vi "EMI_project_v6.vi"() -> ()   [LabVIEW 2020]
uses:
  <vilib>/Instr/_visa.llb/VISA Flush IO Buffer Mask.ctl
  <vilib>/Analysis/baseanly.llb/Mean (DBL).vi
  <vilib>/Instr/_visa.llb/VISA Configure Serial Port (Instr).vi
  <vilib>/Analysis/NI_AALBase.lvlib
panel:
  out "Fader Target Level \nCH02":dbl
  out "Fader Target Level \nCH01":dbl
  out "Ref dB Level CH02":dbl
  out "Ref dB Level CH01":dbl
  out "FSR Level":dbl
  out "Voltage Average Per 5s":dbl
  out "Voltage Average Per 5s":dbl
  out "Debug":bool
  out "Auto Mix LED":bool
  in  "stop 4":bool
  in  "stop 3":bool
  out "Vol Ave Per 100 ms":dbl
  out "Vol Ave Per 100 ms":dbl
  in  "Auto Mix ON/OFF":bool
  out "Take Average CH02":bool
  out "Take Average CH01":bool
  in  "Take Average CH 01":bool
  out "Voltage Peak CH02":dynamicdata(graph)
  out "Voltage Peak CH01":dynamicdata(graph)
  in  "stop 2":bool
  out "Voltage Threshould\n CH 2":dbl
  in  "Noise Threshould \nCH02":dbl
  in  "Take Average CH 2":bool
  out "Voltage Threshould\n CH 01":dbl
  in  "Noise Threshould\n CH01":dbl
  out "Fader 02 level":dbl
  out "Fader 01 level":dbl
  out "Gain Knob 02 level":dbl
  out "Gain knob 01 level":dbl
  out "manual mode led":bool
  out "Sound Balance Mode":bool
  in  "Gain Knob 02":dbl(knob) scale=0.0..300.0
  in  "Gain Knob 01":dbl(knob) scale=0.0..300.0
  in  "Fader 02 Slider":dbl(slide) scale=0.0..10.0
  in  "Fader 01 Slider":dbl(slide) scale=0.0..10.0
  out "Fader 02 Max":dbl
  out "Fader 01 Max":dbl
  in  "Calibrate":bool
  in  "stop":bool
  in  "VISA Resource":refnum<visa-resource-name>
  in  "?":bool
  in  "Gain 02":bool
  in  "?":bool
  in  "Gain 01":bool
  in  "?":bool
  in  "Fader 02":bool
  in  "?":bool
  in  "Fader 01":bool
  # "Automation System For Analog Audio Mixers V 1.0"
  # "Calibration \nMode"
  # "Manual Mode"
  # "Sound Balance Mode"
  # "CH01"
  # "CH02"
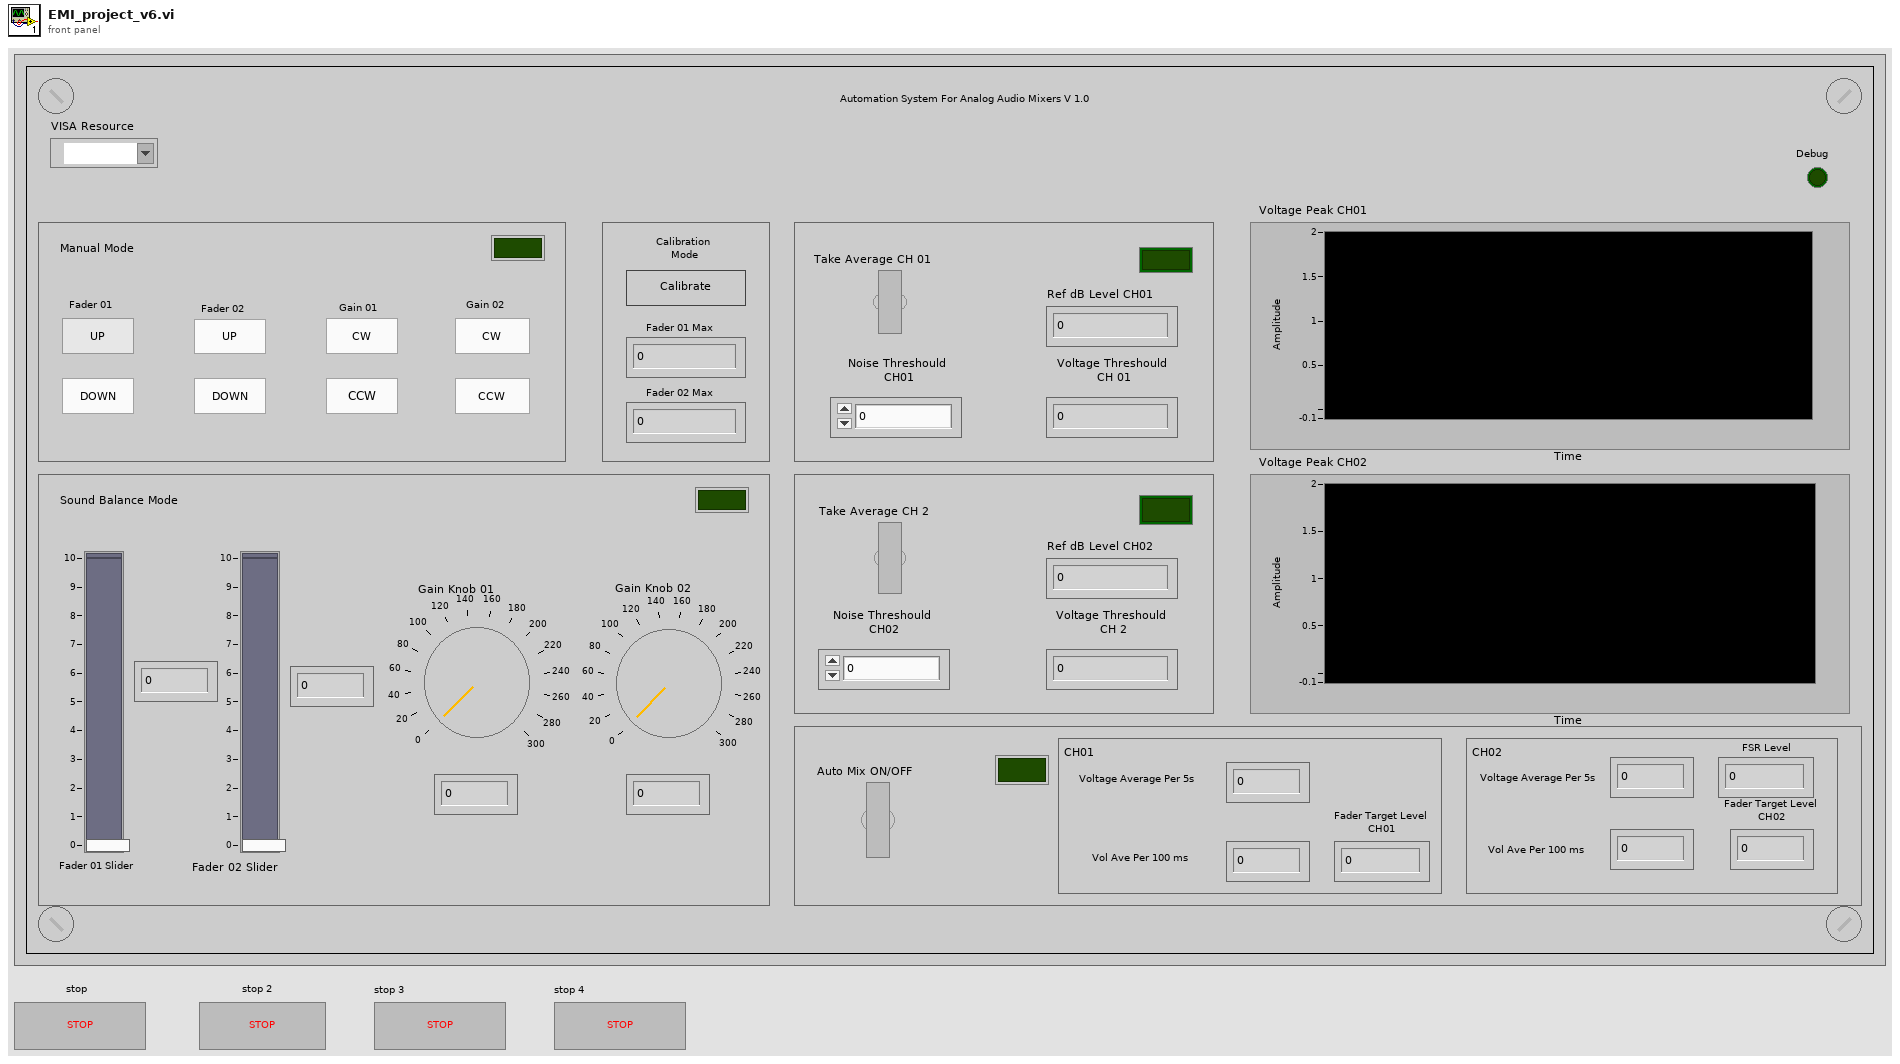
[diagram p1: front panel]
types:
  T1 = cluster{"Fader_Target_mm_1":dbl, "Fader_Target_mm_2":dbl, "Gain_Target_deg_1":dbl, "Gain_Target_deg_2":dbl}
  T2 = typedef "VISA Flush IO Buffer Mask.ctl" = u16
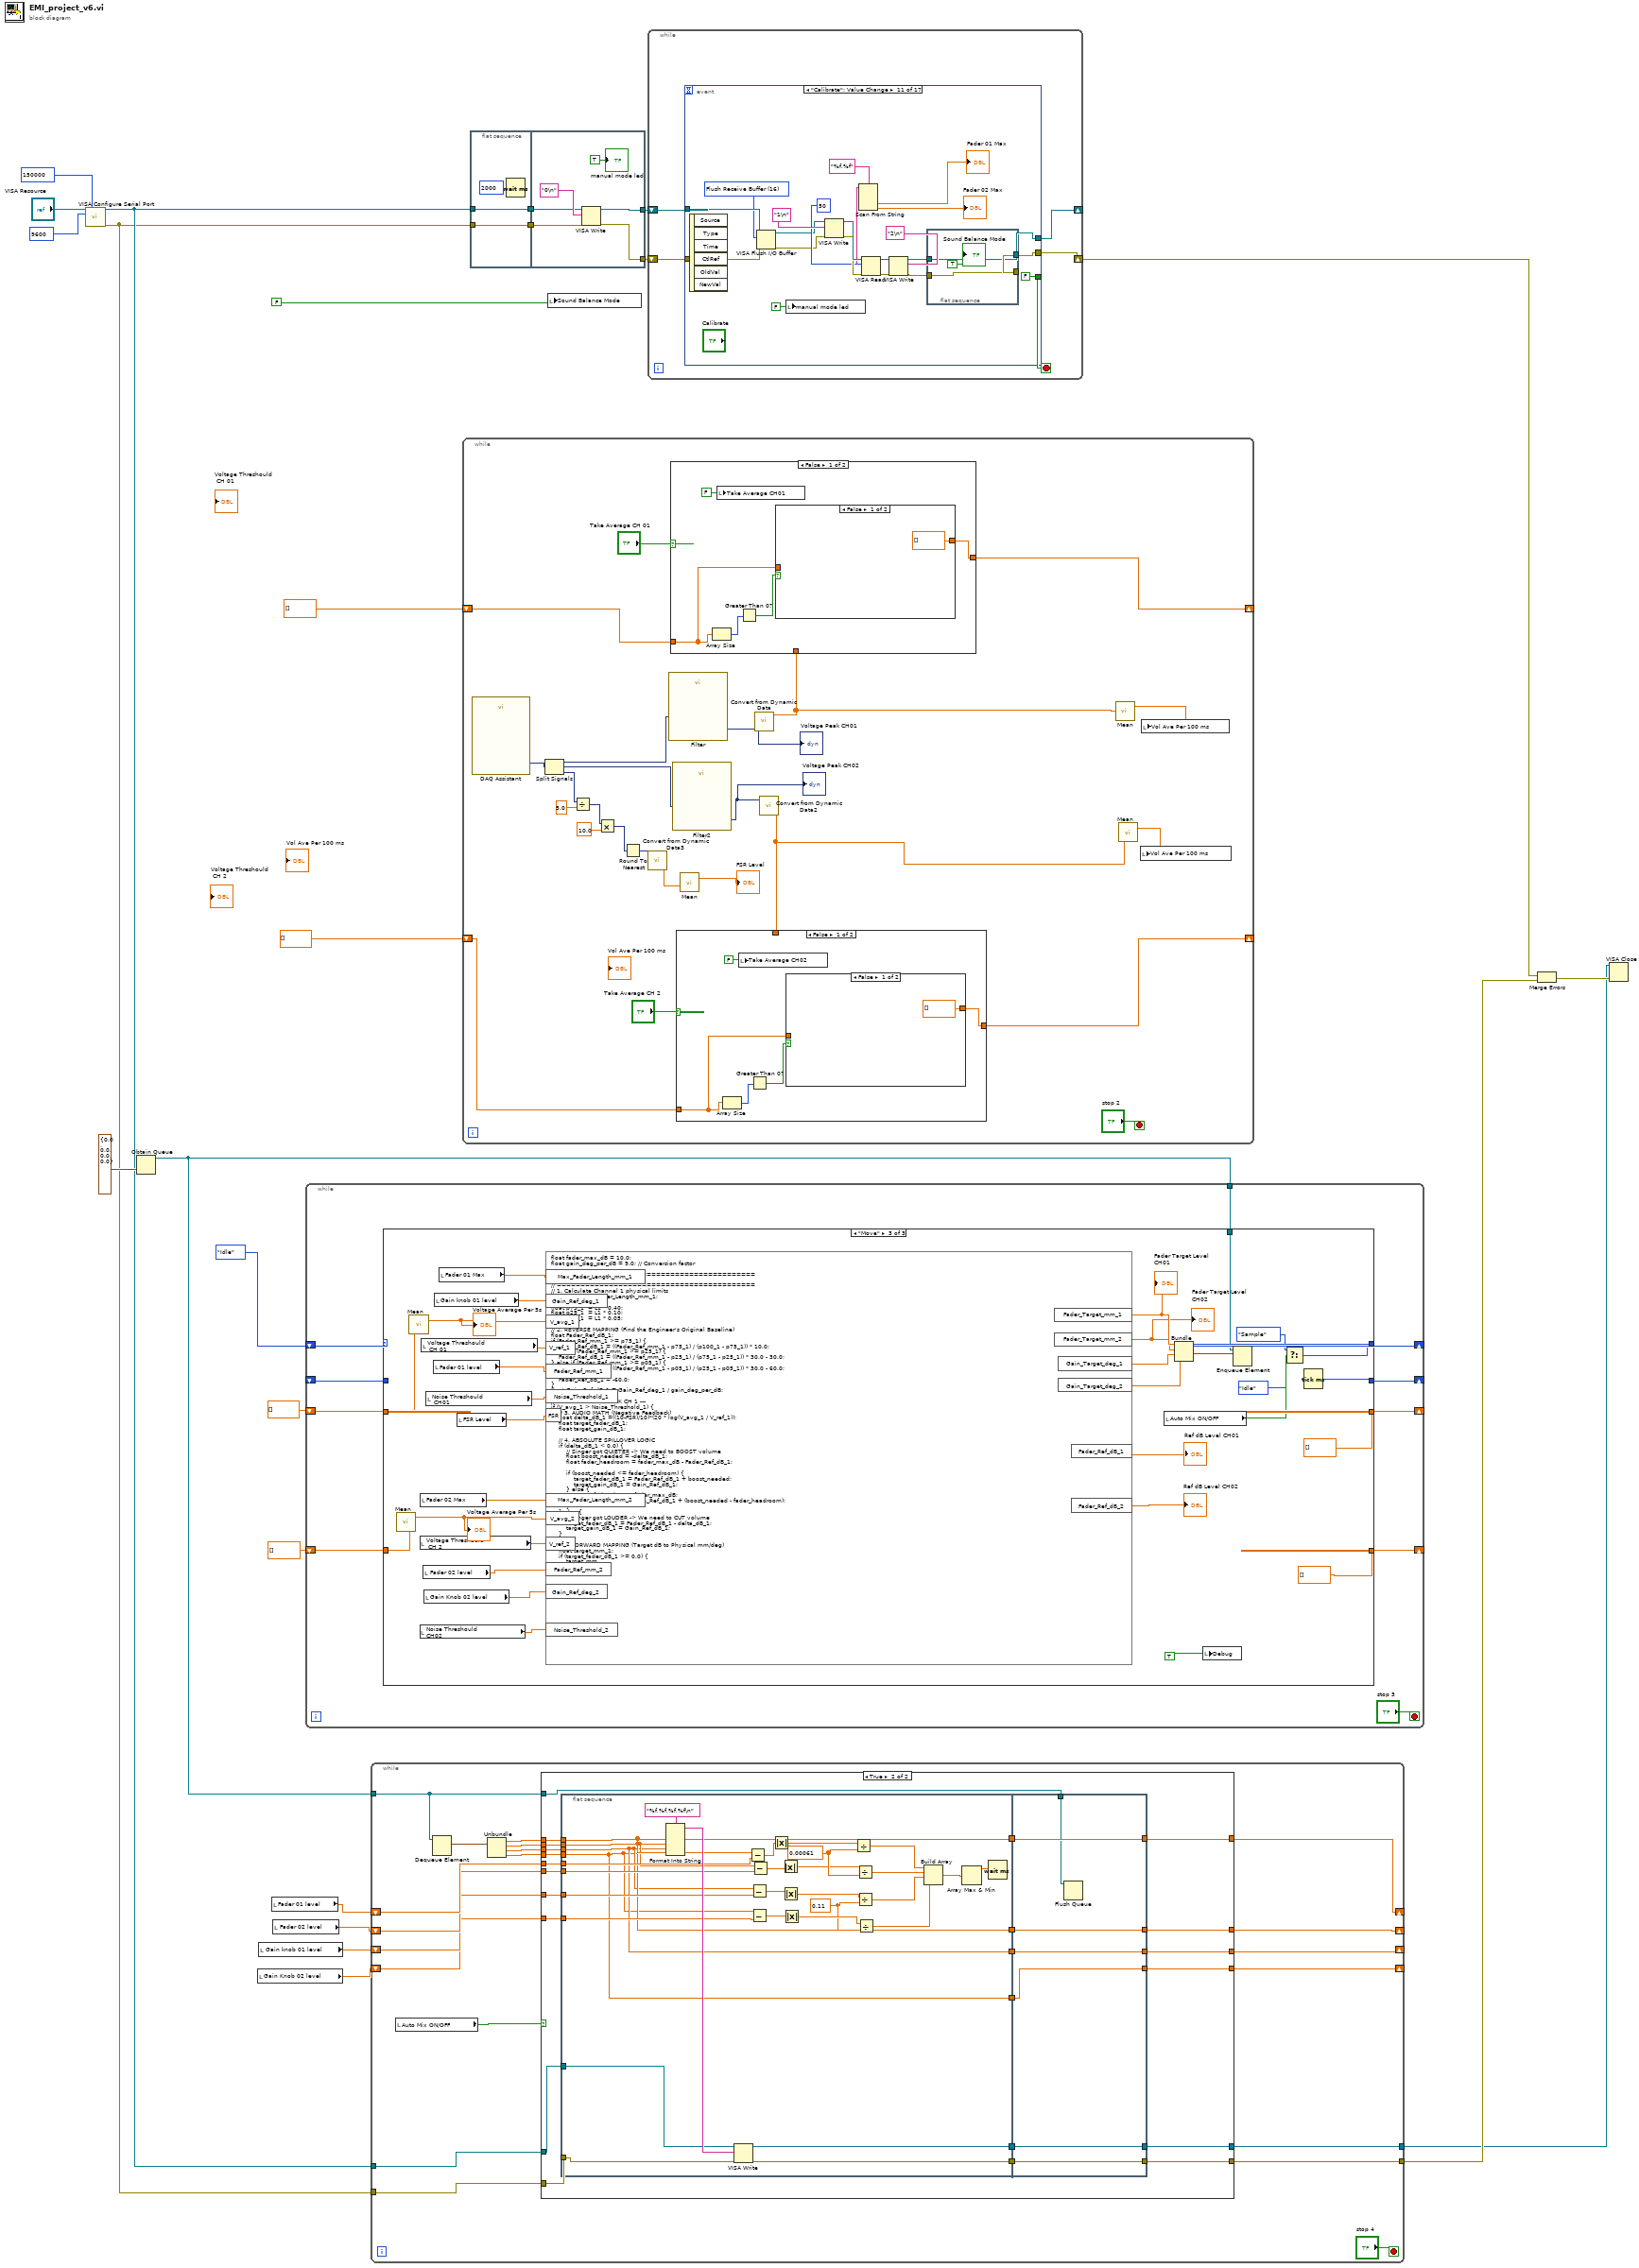
[diagram p0: block diagram]
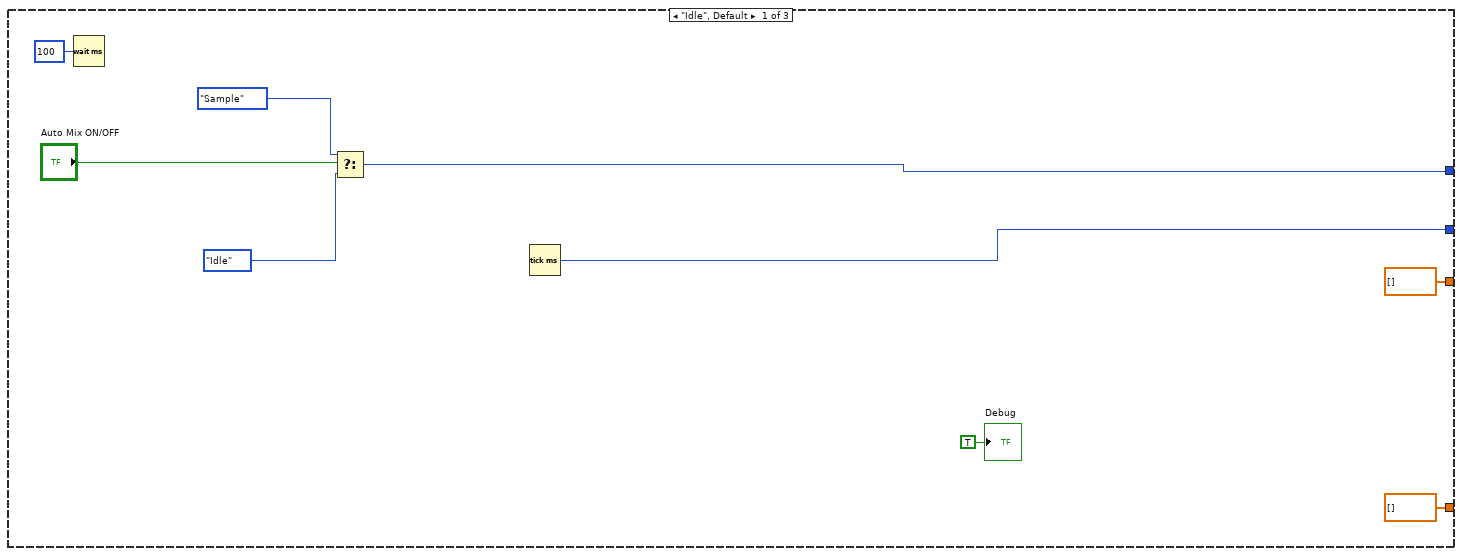
[diagram p3: hidden frame]
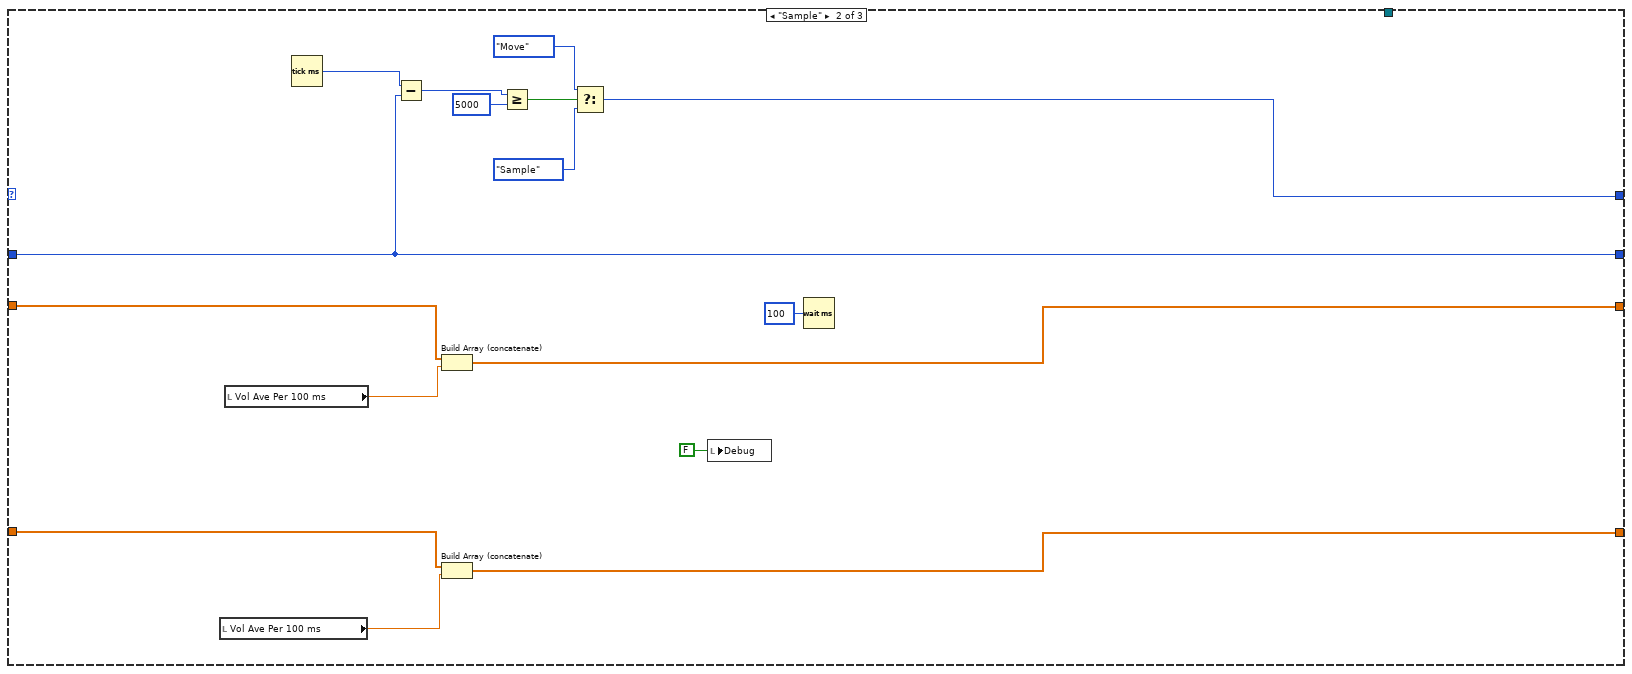
[diagram p4: hidden frame]
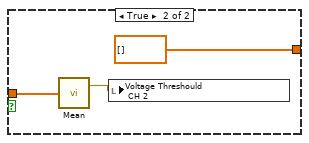
[diagram p5: hidden frame]
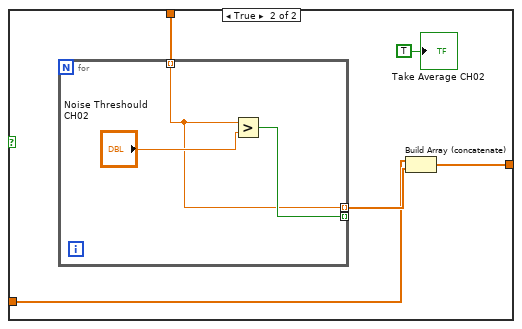
[diagram p6: hidden frame]
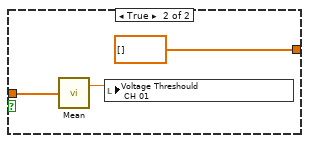
[diagram p7: hidden frame]
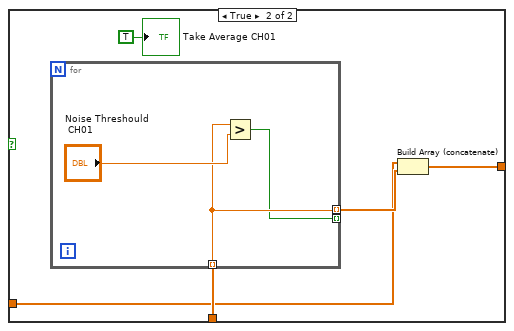
[diagram p8: hidden frame]
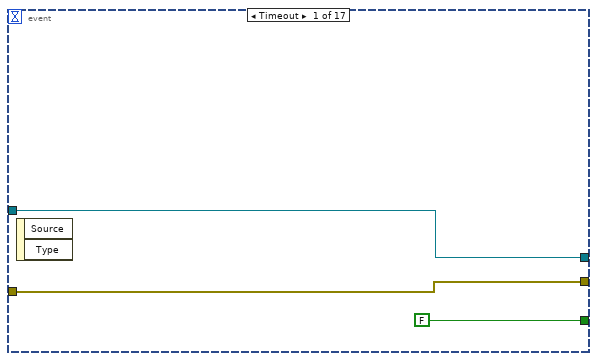
[diagram p9: hidden frame]
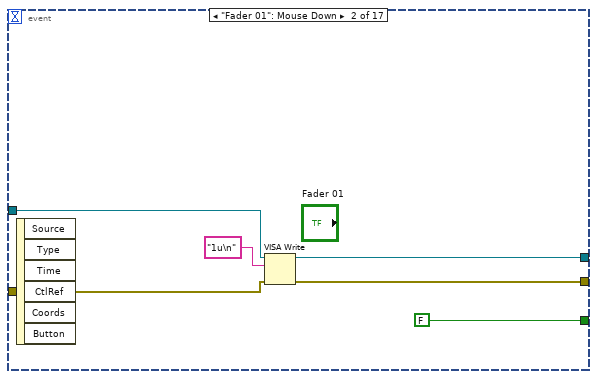
[diagram p10: hidden frame]
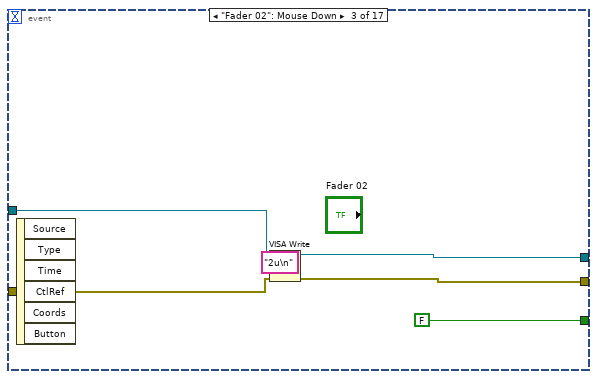
[diagram p11: hidden frame]
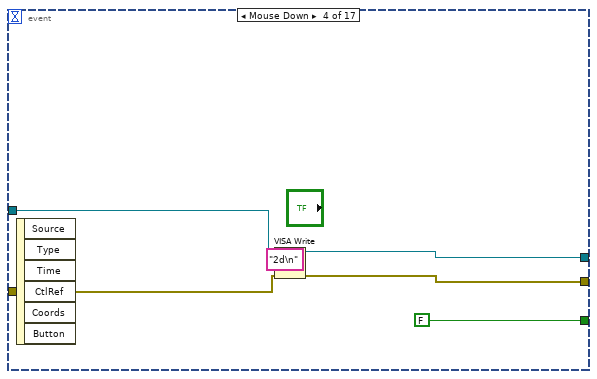
[diagram p12: hidden frame]
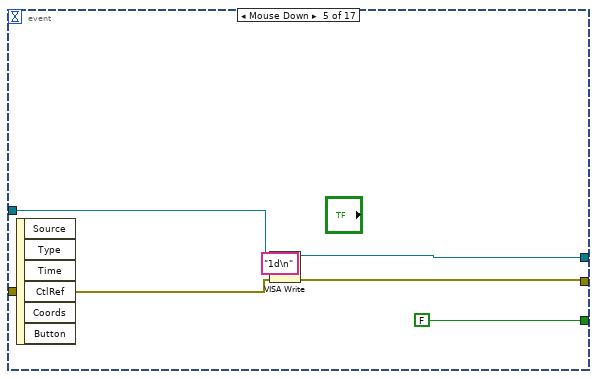
[diagram p13: hidden frame]
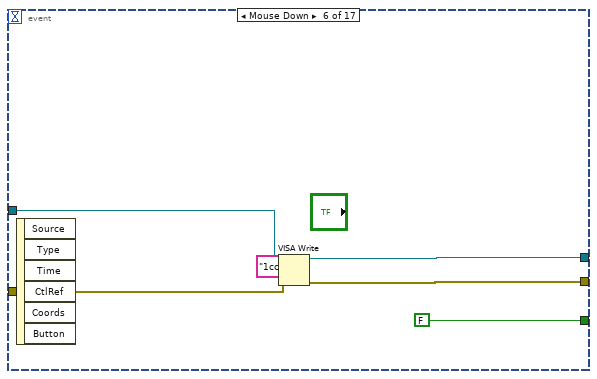
[diagram p14: hidden frame]
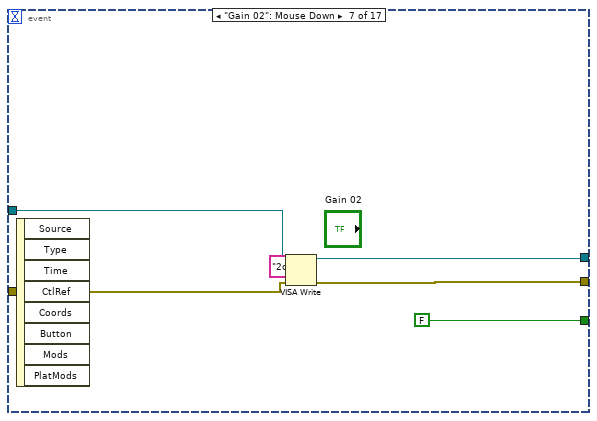
[diagram p15: hidden frame]
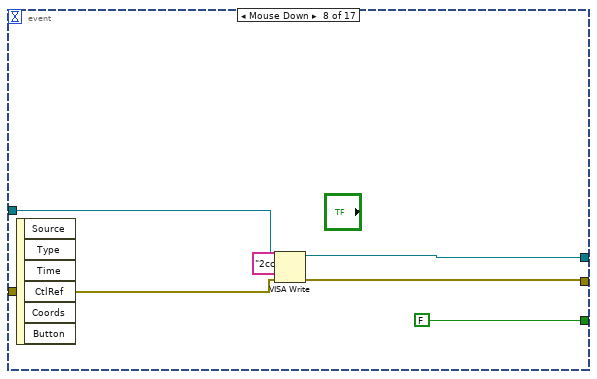
[diagram p16: hidden frame]
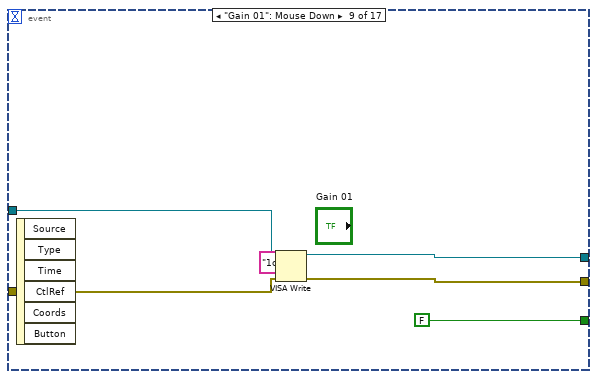
[diagram p17: hidden frame]
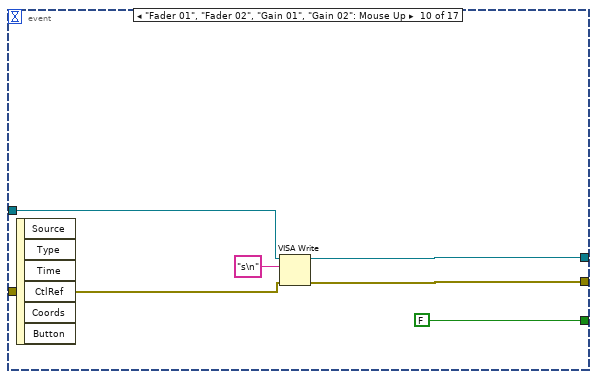
[diagram p18: hidden frame]
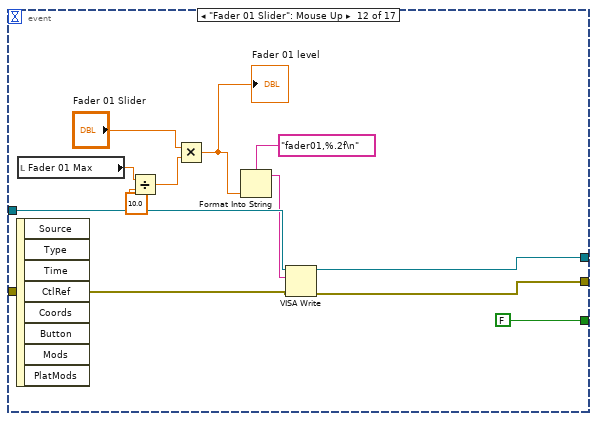
[diagram p19: hidden frame]
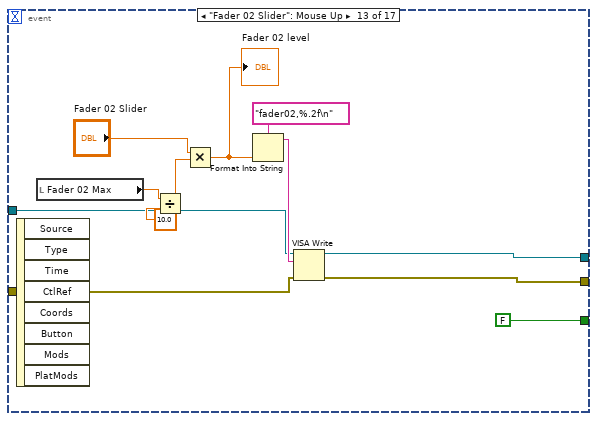
[diagram p20: hidden frame]
diagram:
  n1 = call-poly "VISA Configure Serial Port"("VISA resource name"="VISA Resource", "timeout (10sec)"=u32 150000, "baud rate (9600)"=u32 9600) -> ("VISA resource name out"=w11:refnum<visa-resource-name>, "error out"=w10:errorcluster)  [unwired: 11 in]
  n2 = Obtain Queue(element data type=T1 {"Fader_Target_mm_1"=0.0, "Fader_Target_mm_2"=0.0, "Gain_Target_deg_1"=0.0, "Gain_Target_deg_2"=0.0} ("output cluster")) -> (queue out=w12:refnum<queue>)  [unwired: 4 in, 2 out]
  n3 = local read "Gain Knob 02 level"() -> (w6:dbl)
  n4 = local read "Gain knob 01 level"() -> (w7:dbl)
  n5 = local read "Fader 01 level"() -> (w9:dbl)
  n6 = local read "Fader 02 level"() -> (w8:dbl)
  n7 = while {
    shift-right: [w34] -> _
    shift-left: enum16{"Idle", "Sample", "Move"}."Idle" -> [w35]
    shift-right: [w33] -> _
    shift-left: _ -> [w32]
    shift-right: [w30] -> _
    shift-left: dbl[] [] -> [w31]
    shift-right: [w29] -> _
    shift-left: dbl[] [] -> [w28]
    tunnel: w12 -> [w26]
    stop <- "stop 3" stop-if-true
    n8 = case shown="\"Move\"" w35 {
      tunnel: [w41 w54 w74] -> w34
      tunnel: [w36 w58 w69] -> w33
      tunnel: w32 -> [_ w58 _]
      tunnel: w31 -> [_ w53 w91]
      tunnel: [dbl[] [] w51 dbl[] []] -> w30
      tunnel: [dbl[] [] w48 dbl[] []] -> w29
      tunnel: w28 -> [_ w47 w88]
      tunnel: w26 -> [_ _ w79]
      frame "Idle", Default {
        n9 = Wait (ms)(milliseconds to wait=u32 100) -> ()  [unwired: 1 out]
        n10 = Select(t=enum16{"Idle", "Sample", "Move", "Wait"}."Sample", s="Auto Mix ON/OFF", f=enum16{"Idle", "Sample", "Move", "Wait"}."Idle") -> (s? t:f=w41:enum16{"Idle", "Sample", "Move", "Wait"})
        n11 = Tick Count (ms)() -> (millisecond timer value=w36:u32)
        "Debug" <- TRUE ("Boolean")
      }
      frame "Sample" {
        n12 = local read "Vol Ave Per 100 ms"() -> (w49:dbl)
        n13 = local read "Vol Ave Per 100 ms"() -> (w52:dbl)
        n14 = Tick Count (ms)() -> (millisecond timer value=w45:u32)
        n15 = Subtract(x=w45, y=w58) -> (x-y=w60:u32)
        n16 = Build Array (concatenate)(w53, w52) -> (w51:dbl[])
        n17 = Build Array (concatenate)(w47, w49) -> (w48:dbl[])
        n18 = Greater Or Equal?(x=w60, y=u32 5000) -> (x >= y?=w57:bool)
        n19 = Select(t=enum16{"Idle", "Sample", "Move", "Wait"}."Move", s=w57, f=enum16{"Idle", "Sample", "Move", "Wait"}."Sample") -> (s? t:f=w54:enum16{"Idle", "Sample", "Move", "Wait"})
        n20 = local write "Debug"(FALSE ("Boolean")) -> ()
        n21 = Wait (ms)(milliseconds to wait=u32 100) -> ()  [unwired: 1 out]
      }
      frame "Move" {
        n22 = call-poly <vilib>:"Mean.vi"("X"=w88) -> ("mean"=w67:dbl)  [unwired: 1 out]
        "Voltage Average Per 5s" <- w67
        n23 = call-poly <vilib>:"Mean.vi"("X"=w91) -> ("mean"=w68:dbl)  [unwired: 1 out]
        "Voltage Average Per 5s" <- w68
        n24 = local read "Voltage Threshould\n CH 2"() -> (w85:dbl)
        n25 = local read "Noise Threshould \nCH02"() -> (w71:dbl)
        n26 = local read "Fader 02 Max"() -> (w73:dbl)
        n27 = local read "Voltage Threshould\n CH 01"() -> (w86:dbl)
        n28 = local read "Fader 02 level"() -> (w82:dbl)
        n29 = local read "Gain Knob 02 level"() -> (w81:dbl)
        n30 = local read "Noise Threshould\n CH01"() -> (w72:dbl)
        n31 = local read "Fader 01 level"() -> (w84:dbl)
        n32 = local read "Gain knob 01 level"() -> (w83:dbl)
        n33 = local read "Fader 01 Max"() -> (w87:dbl)
        n34 = local read "FSR Level"() -> (w66:dbl)
        n35 = formula code="float fader_max_dB = 10.0;\nfloat gain_deg_per_dB = 9.0; // Conversion factor\n\n// ==========================================\n// CHANNEL 1 PROCESSING\n// ==========================================\n// 1. Calculate Channel 1 physical limits\nfloat L1 = Max_Fader_Length_mm_1; \nfloat p100_1 = L1;           \nfloat p75_1  = L1 * 0.40;    \nfloat p25_1  = L1 * 0.10;    \nfloat p05_1  = L1 * 0.05;    \n\n// 2. REVERSE MAPPING (Find the Engineer's Original Baseline)\nfloat Fader_Ref_dB_1;\nif (Fader_Ref_mm_1 >= p75_1) {\n    Fader_Ref_dB_1 = ((Fader_Ref_mm_1 - p75_1) / (p100_1 - p75_1)) * 10.0;\n} else if (Fader_Ref_mm_1 >= p25_1) {\n    Fader_Ref_dB_1 = ((Fader_Ref_mm_1 - p25_1) / (p75_1 - p25_1)) * 30.0 - 30.0;\n} else if (Fader_Ref_mm_1 >= p05_1) {\n    Fader_Ref_dB_1 = ((Fader_Ref_mm_1 - p05_1) / (p25_1 - p05_1)) * 30.0 - 60.0;\n} else {\n    Fader_Ref_dB_1 = -60.0; \n}\nfloat Gain_Ref_dB_1 = Gain_Ref_deg_1 / gain_deg_per_dB;\n\n// --- NOISE GATE CHECK CH 1 ---\nif (V_avg_1 > Noise_Threshold_1) {\n    // 3. AUDIO MATH (Negative Feedback)\n    float delta_dB_1 =((10-FSR)/10)*(20 * log(V_avg_1 / V_ref_1));\n    float target_fader_dB_1;\n    float target_gain_dB_1;\n\n    // 4. ABSOLUTE SPILLOVER LOGIC\n    if (delta_dB_1 < 0.0) {\n        // Singer got QUIETER -> We need to BOOST volume\n        float boost_needed = -delta_dB_1; \n        float fader_headroom = fader_max_dB - Fader_Ref_dB_1;\n        \n        if (boost_needed <= fader_headroom) {\n            target_fader_dB_1 = Fader_Ref_dB_1 + boost_needed;\n            target_gain_dB_1 = Gain_Ref_dB_1;\n        } else {\n            target_fader_dB_1 = fader_max_dB;\n            target_gain_dB_1 = Gain_Ref_dB_1 + (boost_needed - fader_headroom);\n        }\n    } else {\n        // Singer got LOUDER -> We need to CUT volume\n        target_fader_dB_1 = Fader_Ref_dB_1 - delta_dB_1;\n        target_gain_dB_1 = Gain_Ref_dB_1;\n    }\n\n    // 5. FORWARD MAPPING (Target dB to Physical mm/deg)\n    float target_mm_1;\n    if (target_fader_dB_1 >= 0.0) {\n        target_mm_1 = p75_1 + ((target_fader_dB_1 - 0.0) / 10.0) * (p100_1 - p75_1);\n    } else if (target_fader_dB_1 >= -30.0) {\n        target_mm_1 = p25_1 + ((target_fader_dB_1 - (-30.0)) / 30.0) * (p75_1 - p25_1);\n    } else if (target_fader_dB_1 >= -60.0) {\n        target_mm_1 = p05_1 + ((target_fader_dB_1 - (-60.0)) / 30.0) * (p25_1 - p05_1);\n    } else {\n        target_mm_1 = 0.0; \n    }\n\n    Fader_Target_mm_1 = target_mm_1;\n    Gain_Target_deg_1 = target_gain_dB_1 * gain_deg_per_dB; \n\n    // 6. HARDWARE SAFETY CLAMP\n    if (Gain_Target_deg_1 > 300) { Gain_Target_deg_1 = 300; }\n    if (Gain_Target_deg_1 < 0.0) { Gain_Target_deg_1 = 0.0; }\n\n} else {\n    // AUDIO IS BELOW NOISE THRESHOLD\n    // Do nothing: lock the targets to the current physical positions\n    Fader_Target_mm_1 = Fader_Ref_mm_1;\n    Gain_Target_deg_1 = Gain_Ref_deg_1;\n}\n\n\n// ==========================================\n// CHANNEL 2 PROCESSING\n// ==========================================\n// 1. Calculate Channel 2 physical limits\nfloat L2 = Max_Fader_Length_mm_2; \nfloat p100_2 = L2;           \nfloat p75_2  = L2 * 0.50;    \nfloat p25_2  = L2 * 0.10;    \nfloat p05_2  = L2 * 0.05;    \n\n// 2. REVERSE MAPPING (Find the Engineer's Original Baseline)\nfloat Fader_Ref_dB_2;\nif (Fader_Ref_mm_2 >= p75_2) {\n    Fader_Ref_dB_2 = ((Fader_Ref_mm_2 - p75_2) / (p100_2 - p75_2)) * 10.0;\n} else if (Fader_Ref_mm_2 >= p25_2) {\n    Fader_Ref_dB_2 = ((Fader_Ref_mm_2 - p25_2) / (p75_2 - p25_2)) * 30.0 - 30.0;\n} else if (Fader_Ref_mm_2 >= p05_2) {\n    Fader_Ref_dB_2 = ((Fader_Ref_mm_2 - p05_2) / (p25_2 - p05_2)) * 30.0 - 60.0;\n} else {\n    Fader_Ref_dB_2 = -60.0; \n}\nfloat Gain_Ref_dB_2 = Gain_Ref_deg_2 / gain_deg_per_dB;\n\n// --- NOISE GATE CHECK CH 2 ---\nif (V_avg_2 > Noise_Threshold_2) {\n    // 3. AUDIO MATH (Negative Feedback)\n    float delta_dB_2 = 20 * log(V_avg_1 / V_ref_1);\n    float target_fader_dB_2;\n    float target_gain_dB_2;\n\n    // 4. ABSOLUTE SPILLOVER LOGIC\n    if (delta_dB_2 < 0.0) {\n        // Singer got QUIETER -> We need to BOOST volume\n        float boost_needed = -delta_dB_2; \n        float fader_headroom = fader_max_dB - Fader_Ref_dB_2;\n        \n        if (boost_needed <= fader_headroom) {\n            target_fader_dB_2 = Fader_Ref_dB_2 + boost_needed;\n            target_gain_dB_2 = Gain_Ref_dB_2;\n        } else {\n            target_fader_dB_2 = fader_max_dB;\n            target_gain_dB_2 = Gain_Ref_dB_2 + (boost_needed - fader_headroom);\n        }\n    } else {\n        // Singer got LOUDER -> We need to CUT volume\n        target_fader_dB_2 = Fader_Ref_dB_2 - delta_dB_2;\n        target_gain_dB_2 = Gain_Ref_dB_2;\n    }\n\n    // 5. FORWARD MAPPING (Target dB to Physical mm/deg)\n    float target_mm_2;\n    if (target_fader_dB_2 >= 0.0) {\n        target_mm_2 = p75_2 + ((target_fader_dB_2 - 0.0) / 10.0) * (p100_2 - p75_2);\n    } else if (target_fader_dB_2 >= -30.0) {\n        target_mm_2 = p25_2 + ((target_fader_dB_2 - (-30.0)) / 30.0) * (p75_2 - p25_2);\n    } else if (target_fader_dB_2 >= -60.0) {\n        target_mm_2 = p05_2 + ((target_fader_dB_2 - (-60.0)) / 30.0) * (p25_2 - p05_2);\n    } else {\n        target_mm_2 = 0.0; \n    }\n\n    Fader_Target_mm_2 = target_mm_2;\n    Gain_Target_deg_2 = target_gain_dB_2 * gain_deg_per_dB; \n\n    // 6. HARDWARE SAFETY CLAMP\n    if (Gain_Target_deg_2 > 300) { Gain_Target_deg_2 = 300; }\n    if (Gain_Target_deg_2 < 0.0) { Gain_Target_deg_2 = 0.0; }\n\n} else {\n    // AUDIO IS BELOW NOISE THRESHOLD\n    // Do nothing: lock the targets to the current physical positions\n    Fader_Target_mm_2 = Fader_Ref_mm_2;\n    Gain_Target_deg_2 = Gain_Ref_deg_2;\n}"("Max_Fader_Length_mm_1"=w87, "Max_Fader_Length_mm_2"=w73, "V_avg_1"=w68, "V_ref_1"=w86, "V_avg_2"=w67, "V_ref_2"=w85, "Fader_Ref_mm_1"=w84, "Fader_Ref_mm_2"=w82, "Gain_Ref_deg_1"=w83, "Gain_Ref_deg_2"=w81, "Noise_Threshold_1"=w72, "Noise_Threshold_2"=w71, "FSR"=w66) -> ("Fader_Target_mm_1"=w63:dbl, "Fader_Target_mm_2"=w61:dbl, "Gain_Target_deg_1"=w80:dbl, "Gain_Target_deg_2"=w62:dbl, "Fader_Ref_dB_1"=→"Ref dB Level CH01":dbl, "Fader_Ref_dB_2"=→"Ref dB Level CH02":dbl)
        "Fader Target Level \nCH01" <- w63
        "Fader Target Level \nCH02" <- w61
        n36 = local read "Auto Mix ON/OFF"() -> (w77:bool)
        n37 = Bundle("Fader_Target_mm_1"=w63, "Fader_Target_mm_2"=w61, "Gain_Target_deg_1"=w80, "Gain_Target_deg_2"=w62) -> (w78:T1)  [unwired: 1 in]
        n38 = local write "Debug"(TRUE ("Boolean")) -> ()
        n39 = Enqueue Element(queue=w79, element=w78) -> ()  [unwired: 2 in, 3 out]
        n40 = Select(t=enum16{"Idle", "Sample", "Move", "Wait"}."Sample", s=w77, f=enum16{"Idle", "Sample", "Move", "Wait"}."Idle") -> (s? t:f=w74:enum16{"Idle", "Sample", "Move", "Wait"})
        n41 = Tick Count (ms)() -> (millisecond timer value=w69:u32)
      }
    }
  }
  n42 = while {
    tunnel: w12 -> [w92]
    tunnel: w11 -> [w105]
    tunnel: w10 -> [w104]
    shift-right: [w99] -> _
    shift-left: w9 -> [w103]
    shift-right: [w98] -> _
    shift-left: w8 -> [w102]
    shift-right: [w97] -> _
    shift-left: w7 -> [w101]
    shift-right: [w96] -> _
    shift-left: w6 -> [w100]
    tunnel: [w95] -> w2
    tunnel: [w94] -> w5
    stop <- "stop 4" stop-if-true
    n43 = local read "Auto Mix ON/OFF"() -> (w110:bool)
    n44 = Dequeue Element(queue=w92) -> (element=w111:T1)  [unwired: 2 in, 3 out]
    n45 = Unbundle(w111) -> ("Fader_Target_mm_1"=w109:dbl, "Fader_Target_mm_2"=w108:dbl, "Gain_Target_deg_1"=w107:dbl, "Gain_Target_deg_2"=w106:dbl)
    n46 = case shown="True" w110 {
      tunnel: w109 -> [_ w140]
      tunnel: w108 -> [_ w139]
      tunnel: w107 -> [_ w138]
      tunnel: w106 -> [_ w137]
      tunnel: w105 -> [w113 w135]
      tunnel: w104 -> [w112 w136]
      tunnel: w103 -> [w117 w134]
      tunnel: w102 -> [w116 w133]
      tunnel: w101 -> [w115 w132]
      tunnel: w100 -> [w114 w131]
      tunnel: [w117 w129] -> w99
      tunnel: [w116 w128] -> w98
      tunnel: [w115 w126] -> w97
      tunnel: [w114 w123] -> w96
      tunnel: [w113 w122] -> w95
      tunnel: [w112 w120] -> w94
      tunnel: w92 -> [_ w118]
      frame False {
      }
      frame True {
        n47 = flat-sequence {
          tunnel: w140 -> [w148]
          tunnel: w139 -> [w147]
          tunnel: w138 -> [w146]
          tunnel: w137 -> [w145]
          tunnel: w136 -> [w141]
          tunnel: w135 -> [w142]
          tunnel: w134 -> [w168]
          tunnel: w133 -> [w167]
          tunnel: w132 -> [w166]
          tunnel: w131 -> [w165]
          tunnel: [w148] -> w130
          tunnel: [w147] -> w127
          tunnel: [w146] -> w125
          tunnel: [w145] -> w124
          tunnel: [w144] -> w121
          tunnel: [w143] -> w119
          tunnel: w130 -> [w177]
          tunnel: [w177] -> w129
          tunnel: [w176] -> w128
          tunnel: w127 -> [w176]
          tunnel: [w175] -> w126
          tunnel: w125 -> [w175]
          tunnel: w124 -> [w174]
          tunnel: [w174] -> w123
          tunnel: [w173] -> w122
          tunnel: w121 -> [w173]
          tunnel: [w172] -> w120
          tunnel: w119 -> [w172]
          tunnel: w118 -> [w171]
          frame #0 {
            w151 = 0.11 ("y")
            w160 = 0.00061 ("y")
            n48 = Format Into String(format string="%f,%f,%f,%f\n", w148, w147, w146, w145) -> (resulting string=w169:string)  [unwired: 2 in, 1 out]
            n49 = VISA Write(VISA resource name=w142, write buffer=w169, error in (no error)=w141) -> (VISA resource name out=w144:refnum<visa-resource-name>, error out=w143:errorcluster)  [unwired: 1 out]
            n50 = Subtract(x=w148, y=w168) -> (x-y=w164:dbl)
            n51 = Subtract(x=w146, y=w166) -> (x-y=w162:dbl)
            n52 = Subtract(x=w145, y=w165) -> (x-y=w161:dbl)
            n53 = Subtract(x=w147, y=w167) -> (x-y=w163:dbl)
            n54 = Absolute Value(x=w164) -> (abs(x)=w159:dbl)
            n55 = Absolute Value(x=w163) -> (abs(x)=w158:dbl)
            n56 = Absolute Value(x=w162) -> (abs(x)=w157:dbl)
            n57 = Absolute Value(x=w161) -> (abs(x)=w156:dbl)
            n58 = Divide(x=w159, y=w160) -> (x/y=w155:dbl)
            n59 = Divide(x=w158, y=w160) -> (x/y=w154:dbl)
            n60 = Divide(x=w157, y=w151) -> (x/y=w153:dbl)
            n61 = Divide(x=w156, y=w151) -> (x/y=w152:dbl)
            n62 = Build Array(w155, w154, w153, w152) -> (w150:dbl[])
            n63 = Array Max & Min(array=w150) -> (max value=w149:dbl)  [unwired: 3 out]
            n64 = Wait (ms)(milliseconds to wait=w149) -> ()  [unwired: 1 out]
          }
          frame #1 {
            n65 = Flush Queue(queue=w171) -> ()  [unwired: 1 in, 3 out]
          }
        }
      }
    }
  }
  n66 = while {
    shift-right: [w197] -> _
    shift-left: dbl[] [] -> [w198]
    shift-right: [w195] -> _
    shift-left: dbl[] [] -> [w194]
    stop <- "stop 2" stop-if-true
    n67 = call "DAQ Assistant"() -> ("data"=w186:dynamicdata)  [unwired: 16 in, 3 out]
    n68 = Split Signals(w186) -> (w200:dynamicdata, w199:dynamicdata, w178:dynamicdata)  [unwired: 3 in]
    n69 = Divide(x=w178, y=5.0) -> (x/y=w183:dynamicdata)
    n70 = Multiply(x=w183, y=10.0) -> (x*y=w180:dynamicdata)
    n71 = Round To Nearest(number=w180) -> (nearest integer value=w179:dynamicdata)
    n72 = call "Convert from Dynamic Data3"("Dynamic Data Type"=w179) -> ("Array"=w184:dbl[])  [unwired: 3 in]
    n73 = call "Filter"("Signal"=w200) -> ("Filtered Signal"=w192:dynamicdata)  [unwired: 9 in, 1 out]
    "Voltage Peak CH01" <- w192
    n74 = call "Filter2"("Signal"=w199) -> ("Filtered Signal"=w191:dynamicdata)  [unwired: 9 in, 1 out]
    "Voltage Peak CH02" <- w191
    n75 = call-poly <vilib>:"Mean.vi"("X"=w184) -> ("mean"=→"FSR Level":dbl)  [unwired: 1 out]
    n76 = call "Convert from Dynamic Data"("Dynamic Data Type"=w192) -> ("Array"=w188:dbl[])  [unwired: 3 in]
    n77 = case shown="False" "Take Average CH 01" {
      tunnel: w188 -> [_ w232]
      tunnel: w198 -> [w221 w229]
      tunnel: [w220 w230] -> w197
      frame False {
        n78 = Array Size(array=w221) -> (size(s)=w223:i32)
        n79 = local write "Take Average CH01"(FALSE ("Take Average CH01")) -> ()
        n80 = Greater Than 0?(x=w223) -> (x > 0?=w222:bool)
        n81 = case shown="False" w222 {
          tunnel: w221 -> [_ w227]
          tunnel: [dbl[] [] dbl[] []] -> w220
          frame False {
          }
          frame True {
            n82 = call-poly <vilib>:"Mean.vi"("X"=w227) -> ("mean"=w226:dbl)  [unwired: 1 out]
            n83 = local write "Voltage Threshould\n CH 01"(w226) -> ()
          }
        }
      }
      frame True {
        n84 = for {
          tunnel: w232 -> [w234] mode=indexing
          tunnel: [w234] -> w231 mode=indexing if=w233
          tunnel: [w233] -> _ mode=indexing
          n85 = Greater?(x=w234, y="Noise Threshould\n CH01") -> (0:w233:bool)
        }
        n86 = Build Array (concatenate)(w229, w231) -> (w230:dbl[])
        "Take Average CH01" <- TRUE ("Take Average CH01")
      }
    }
    n87 = call "Convert from Dynamic Data2"("Dynamic Data Type"=w191) -> ("Array"=w187:dbl[])  [unwired: 3 in]
    n88 = case shown="False" "Take Average CH 2" {
      tunnel: w194 -> [w204 w214]
      tunnel: [w203 w213] -> w195
      tunnel: w187 -> [_ w212]
      frame False {
        n89 = Array Size(array=w204) -> (size(s)=w206:i32)
        n90 = local write "Take Average CH02"(FALSE ("Take Average CH02")) -> ()
        n91 = Greater Than 0?(x=w206) -> (x > 0?=w205:bool)
        n92 = case shown="False" w205 {
          tunnel: w204 -> [_ w210]
          tunnel: [dbl[] [] dbl[] []] -> w203
          frame False {
          }
          frame True {
            n93 = call-poly <vilib>:"Mean.vi"("X"=w210) -> ("mean"=w209:dbl)  [unwired: 1 out]
            n94 = local write "Voltage Threshould\n CH 2"(w209) -> ()
          }
        }
      }
      frame True {
        n95 = for {
          tunnel: [w216] -> w215 mode=indexing if=w217
          tunnel: [w217] -> _ mode=indexing
          tunnel: w212 -> [w216] mode=indexing
          n96 = Greater?(x=w216, y="Noise Threshould \nCH02") -> (0:w217:bool)
        }
        n97 = Build Array (concatenate)(w214, w215) -> (w213:dbl[])
        "Take Average CH02" <- TRUE ("Take Average CH02")
      }
    }
    n98 = call-poly <vilib>:"Mean.vi"("X"=w188) -> ("mean"=w190:dbl)  [unwired: 1 out]
    n99 = call-poly <vilib>:"Mean.vi"("X"=w187) -> ("mean"=w189:dbl)  [unwired: 1 out]
    n100 = local write "Vol Ave Per 100 ms"(w189) -> ()
    n101 = local write "Vol Ave Per 100 ms"(w190) -> ()
  }
  n102 = flat-sequence {
    tunnel: w10 -> [w237]
    tunnel: w11 -> [w238]
    tunnel: [w238] -> w21
    tunnel: [w237] -> w20
    tunnel: [w243] -> w23
    tunnel: [w242] -> w22
    tunnel: w21 -> [w241]
    tunnel: w20 -> [w240]
    frame #0 {
      n103 = Wait (ms)(milliseconds to wait=u32 2000) -> ()  [unwired: 1 out]
    }
    frame #1 {
      n104 = VISA Write(VISA resource name=w241, write buffer="0\n", error in (no error)=w240) -> (VISA resource name out=w243:refnum<visa-resource-name>, error out=w242:errorcluster)  [unwired: 1 out]
      "manual mode led" <- TRUE
    }
  }
  n105 = local write "Sound Balance Mode"(FALSE) -> ()
  n106 = while {
    shift-right: [w247] -> _
    shift-left: w23 -> [w249]
    shift-right: [w246] -> w4
    shift-left: w22 -> [w248]
    stop <- w245 stop-if-true
    n107 = event shown="[10] \"Calibrate\": Value Change" {
      selector: _ -> [_ _ _ _ _ _ _ _ _ _ _ _ _ _ _ _ _]
      dyn-events: _ -> [_ _ _ _ _ _ _ _ _ _ _ _ _ _ _ _ _]
      timeout: _ -> [_ _ _ _ _ _ _ _ _ _ _ _ _ _ _ _ _]
      tunnel: w249 -> [w252 w258 w262 w268 w276 w279 w286 w292 w298 w304 w320 w338 w349 w362 w369 w375 w393]
      tunnel: w248 -> [w251 w257 w261 w267 w275 w280 w285 w291 w297 w303 w319 w337 w348 w361 w368 w373 w392]
      tunnel: [w252 w255 w264 w270 w273 w282 w288 w294 w300 w306 w311 w334 w346 w359 w366 w374 w393] -> w247
      tunnel: [w251 w254 w263 w269 w274 w281 w287 w293 w299 w305 w308 w336 w347 w360 w367 w372 w392] -> w246
      tunnel: [FALSE FALSE FALSE FALSE FALSE FALSE FALSE FALSE FALSE FALSE FALSE FALSE FALSE FALSE FALSE FALSE TRUE] -> w245
      event Timeout {
        n108 = event-data() -> ()  [unwired: 1 in, 2 out]
      }
      event "Fader 01": Mouse Down {
        n109 = event-data() -> ()  [unwired: 1 in, 6 out]
        n110 = VISA Write(VISA resource name=w258, write buffer="1u\n", error in (no error)=w257) -> (VISA resource name out=w255:refnum<visa-resource-name>, error out=w254:errorcluster)  [unwired: 1 out]
      }
      event "Fader 02": Mouse Down {
        n111 = event-data() -> ()  [unwired: 1 in, 6 out]
        n112 = VISA Write(VISA resource name=w262, write buffer="2u\n", error in (no error)=w261) -> (VISA resource name out=w264:refnum<visa-resource-name>, error out=w263:errorcluster)  [unwired: 1 out]
      }
      event Mouse Down {
        n113 = event-data() -> ()  [unwired: 1 in, 6 out]
        n114 = VISA Write(VISA resource name=w268, write buffer="2d\n", error in (no error)=w267) -> (VISA resource name out=w270:refnum<visa-resource-name>, error out=w269:errorcluster)  [unwired: 1 out]
      }
      event Mouse Down {
        n115 = event-data() -> ()  [unwired: 1 in, 6 out]
        n116 = VISA Write(VISA resource name=w276, write buffer="1d\n", error in (no error)=w275) -> (VISA resource name out=w273:refnum<visa-resource-name>, error out=w274:errorcluster)  [unwired: 1 out]
      }
      event Mouse Down {
        n117 = event-data() -> ()  [unwired: 1 in, 6 out]
        n118 = VISA Write(VISA resource name=w279, write buffer="1ccw\n", error in (no error)=w280) -> (VISA resource name out=w282:refnum<visa-resource-name>, error out=w281:errorcluster)  [unwired: 1 out]
      }
      event "Gain 02": Mouse Down {
        n119 = event-data() -> ()  [unwired: 1 in, 8 out]
        n120 = VISA Write(VISA resource name=w286, write buffer="2cw\n", error in (no error)=w285) -> (VISA resource name out=w288:refnum<visa-resource-name>, error out=w287:errorcluster)  [unwired: 1 out]
      }
      event Mouse Down {
        n121 = event-data() -> ()  [unwired: 1 in, 6 out]
        n122 = VISA Write(VISA resource name=w292, write buffer="2ccw\n", error in (no error)=w291) -> (VISA resource name out=w294:refnum<visa-resource-name>, error out=w293:errorcluster)  [unwired: 1 out]
      }
      event "Gain 01": Mouse Down {
        n123 = event-data() -> ()  [unwired: 1 in, 6 out]
        n124 = VISA Write(VISA resource name=w298, write buffer="1cw\n", error in (no error)=w297) -> (VISA resource name out=w300:refnum<visa-resource-name>, error out=w299:errorcluster)  [unwired: 1 out]
      }
      event "Fader 01", "Fader 02", "Gain 01", "Gain 02": Mouse Up {
        n125 = event-data() -> ()  [unwired: 1 in, 6 out]
        n126 = VISA Write(VISA resource name=w304, write buffer="s\n", error in (no error)=w303) -> (VISA resource name out=w306:refnum<visa-resource-name>, error out=w305:errorcluster)  [unwired: 1 out]
      }
      event "Calibrate": Value Change {
        w316 = T2 16 items=["Flush Receive Buffer"=16, "Write Transmit Buffer to Device"=32, "Flush Receive Buffer (No I/O)"=64, "Flush Transmit Buffer"=128] ("Mask")
        n127 = event-data() -> ()  [unwired: 1 in, 6 out]
        n128 = VISA Flush I/O Buffer(VISA resource name=w320, mask (16)=w316, error in (no error)=w319) -> (VISA resource name out=w318:refnum<visa-resource-name>, error out=w317:errorcluster)
        n129 = local write "manual mode led"(FALSE ("manual mode led")) -> ()
        n130 = VISA Write(VISA resource name=w318, write buffer="1\n", error in (no error)=w317) -> (VISA resource name out=w327:refnum<visa-resource-name>, error out=w326:errorcluster)  [unwired: 1 out]
        n131 = VISA Read(VISA resource name=w327, byte count=u32 50, error in (no error)=w326) -> (VISA resource name out=w315:refnum<visa-resource-name>, read buffer=w324:string, error out=w314:errorcluster)  [unwired: 1 out]
        n132 = Scan From String(format string="%f,%f", input string=w324) -> (output 1=→"Fader 01 Max":dbl, output 2=→"Fader 02 Max":dbl)  [unwired: 4 in, 3 out]
        n133 = VISA Write(VISA resource name=w315, write buffer="2\n", error in (no error)=w314) -> (VISA resource name out=w310:refnum<visa-resource-name>, error out=w309:errorcluster)  [unwired: 1 out]
        n134 = flat-sequence {
          tunnel: [w330] -> w311
          tunnel: w310 -> [w330]
          tunnel: w309 -> [w329]
          tunnel: [w329] -> w308
          frame #0 {
            "Sound Balance Mode" <- TRUE
          }
        }
      }
      event "Fader 01 Slider": Mouse Up {
        n135 = event-data() -> ()  [unwired: 1 in, 8 out]
        n136 = local read "Fader 01 Max"() -> (w342:dbl)
        n137 = Divide(x=w342, y=10.0) -> (x/y=w339:dbl)
        n138 = Multiply(x="Fader 01 Slider", y=w339) -> (x*y=w332:dbl)
        "Fader 01 level" <- w332
        n139 = Format Into String(format string="fader01,%.2f\n", w332) -> (resulting string=w333:string)  [unwired: 2 in, 1 out]
        n140 = VISA Write(VISA resource name=w338, write buffer=w333, error in (no error)=w337) -> (VISA resource name out=w334:refnum<visa-resource-name>, error out=w336:errorcluster)  [unwired: 1 out]
      }
      event "Fader 02 Slider": Mouse Up {
        n141 = event-data() -> ()  [unwired: 1 in, 8 out]
        n142 = local read "Fader 02 Max"() -> (w355:dbl)
        n143 = Divide(x=w355, y=10.0) -> (x/y=w352:dbl)
        n144 = Multiply(x="Fader 02 Slider", y=w352) -> (x*y=w344:dbl)
        "Fader 02 level" <- w344
        n145 = Format Into String(format string="fader02,%.2f\n", w344) -> (resulting string=w350:string)  [unwired: 2 in, 1 out]
        n146 = VISA Write(VISA resource name=w349, write buffer=w350, error in (no error)=w348) -> (VISA resource name out=w346:refnum<visa-resource-name>, error out=w347:errorcluster)  [unwired: 1 out]
      }
      event "Gain Knob 01": Mouse Up {
        n147 = event-data() -> ()  [unwired: 1 in, 8 out]
        n148 = Format Into String(format string="gain01,%.2f\n", "Gain Knob 01") -> (resulting string=w358:string)  [unwired: 2 in, 1 out]
        n149 = VISA Write(VISA resource name=w362, write buffer=w358, error in (no error)=w361) -> (VISA resource name out=w359:refnum<visa-resource-name>, error out=w360:errorcluster)  [unwired: 1 out]
        "Gain knob 01 level" <- "Gain Knob 01"
      }
      event "Gain Knob 02": Mouse Up {
        n150 = event-data() -> ()  [unwired: 1 in, 8 out]
        n151 = Format Into String(format string="gain02,%.2f\n", "Gain Knob 02") -> (resulting string=w370:string)  [unwired: 2 in, 1 out]
        n152 = VISA Write(VISA resource name=w369, write buffer=w370, error in (no error)=w368) -> (VISA resource name out=w366:refnum<visa-resource-name>, error out=w367:errorcluster)  [unwired: 1 out]
        "Gain Knob 02 level" <- "Gain Knob 02"
      }
      event "Auto Mix ON/OFF": Value Change {
        n153 = event-data() -> ()  [unwired: 1 in, 6 out]
        n154 = local read "Auto Mix ON/OFF"() -> (w377:bool)
        n155 = case shown="False" w377 {
          tunnel: w375 -> [w381 w391]
          tunnel: [w383 w390] -> w374
          tunnel: w373 -> [w384 w389]
          tunnel: [w382 w388] -> w372
          frame False {
            n156 = local write "Sound Balance Mode"(TRUE ("Sound Balance Mode")) -> ()
            n157 = VISA Write(VISA resource name=w381, write buffer="2\n", error in (no error)=w384) -> (VISA resource name out=w383:refnum<visa-resource-name>, error out=w382:errorcluster)  [unwired: 1 out]
            n158 = local write "Auto Mix LED"(FALSE ("Auto Mix LED")) -> ()
          }
          frame True {
            n159 = VISA Write(VISA resource name=w391, write buffer="3\n", error in (no error)=w389) -> (VISA resource name out=w390:refnum<visa-resource-name>, error out=w388:errorcluster)  [unwired: 1 out]
            n160 = local write "Sound Balance Mode"(FALSE ("Sound Balance Mode")) -> ()
            "Auto Mix LED" <- TRUE ("Auto Mix LED")
          }
        }
      }
      event "stop": Value Change {
        n161 = event-data() -> ()  [unwired: 1 in, 6 out]
      }
    }
  }
  n162 = Merge Errors(w4, w5) -> (w3:errorcluster)
  n163 = VISA Close(VISA resource name=w2, error in (no error)=w3) -> ()  [unwired: 1 out]
